vi "Library file types.vi"() -> ()   [LabVIEW 2017, in "Palette Menu.lvlib"]
uses:
  <vilib>/Palette API/Palette Menu/Palette Menu.lvlib
panel:
  in  "libtype has default palettes":string[](array[string])=["lvlib", "lvclass", "lvlibp"]
  in  "library types":string[](array[string])=["lvlib", "lvclass", "xnode", "xctl", "lvlibp"]
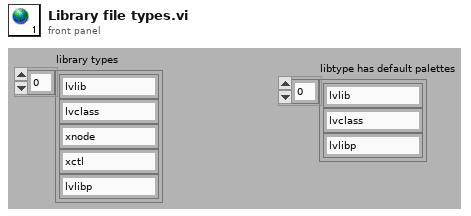
[diagram p1: front panel]
diagram:
